vi "Write ImageDescription to tiff string.vi"(8 "error in":errorcluster, 10 "Tiff image (unsigned byte array)":u8[](array[numeric]), 11 "ImageDescription string\n(must be at least 5 char long)":string) -> (0 "error out":errorcluster, 2 "Tiff file out (unsigned byte array)":u8[](array[numeric]))   [LabVIEW 2015, in "Tiff reader.lvlib"]
doc: "This .vi adds metadata to the tiff file (represented as a string)."
uses:
  Tiff reader.lvlib
  FieldTypes.ctl
  IFD Entry.ctl
panel:
  out "Insert tag before inserting data?":bool
  out "Directories out 2":T1[](array[typedef])
  out "Byte stream offset\nwhere tag should have been":u32
  out "Directories in":T1[](array[typedef])
  out "Val/Offs":u32
  out "Time elapsed (ms)":u32
  out "Tag already exists?":bool
  out "Tag for metadata":T1
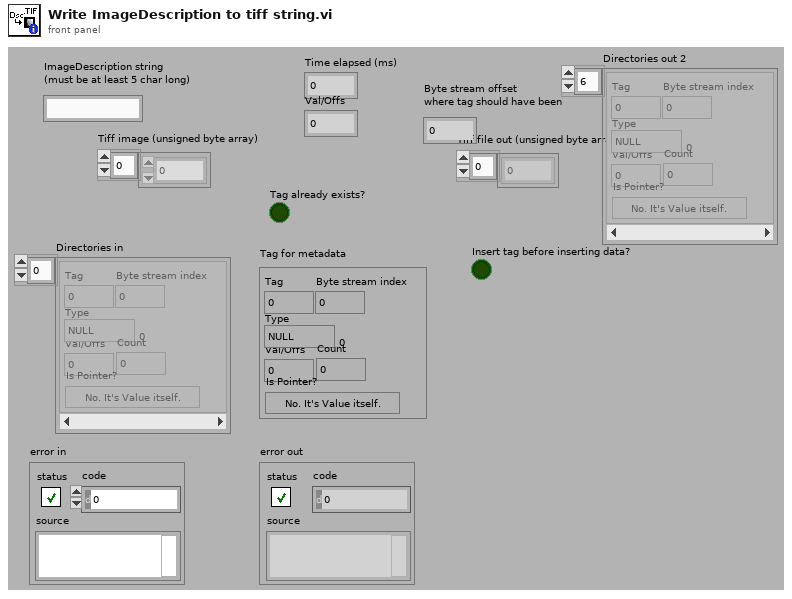
[diagram p1: front panel]
types:
  T1 = typedef "Tiff reader.lvlib/IFD Entry.ctl" = cluster{"Tag":u16, "Type":T2, "Count":u32, "Val/Offs":u32, "Is Pointer?":bool, "Byte stream index":i32}
  T2 = typedef "Tiff reader.lvlib/FieldTypes.ctl" = enum16{"NULL", "U8", "ASCII7", "U16", "U32", "RATIONAL", "SByte(I8)", "Undef(8Bit)", "I16", "I32", "SRat(4B:4B)", "SGL(4Byte)", "DBL(8Byte)"}
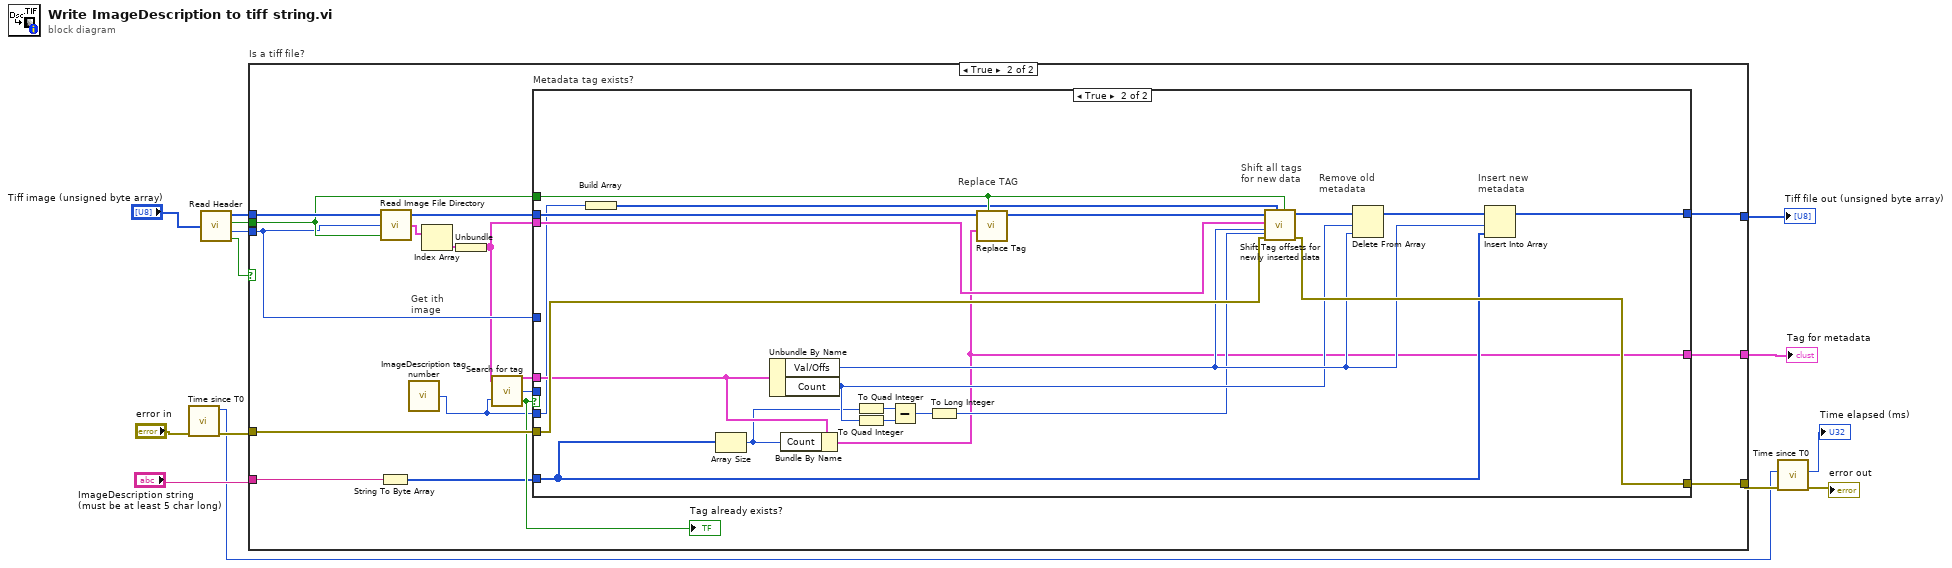
[diagram p0: block diagram]
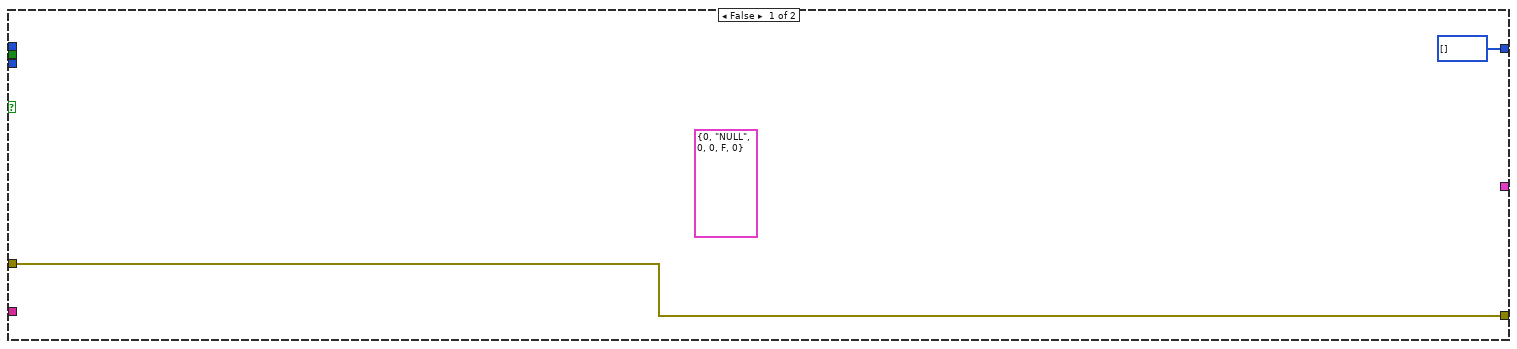
[diagram p2: hidden frame]
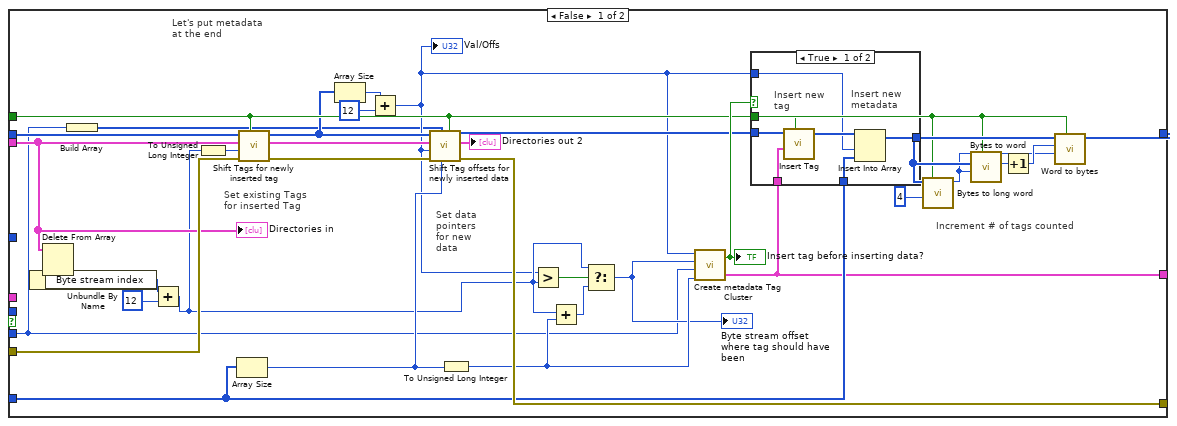
[diagram p3: hidden frame]
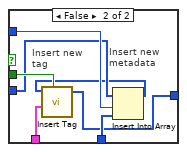
[diagram p4: hidden frame]
diagram:
  n1 = call "Time since T0.vi"("error in (no error)"="error in") -> ("error out"=w7:errorcluster, "current ms"=w3:u32)  [unwired: 2 in, 3 out]
  n2 = call "Read Header.vi"("TIFF Data in"="Tiff image (unsigned byte array)") -> ("TIFF Data out"=w13:u8[], "Litt/BigEnd"=w12:bool, "ImFileDirectOffs"=w14:u32, "IsTIFF?"=w11:bool)
  n3 = case "Is a tiff file?" shown="True" w11 {
    tunnel: w14 -> [_ w27]
    tunnel: w13 -> [_ w29]
    tunnel: [u8[] [] ("Image Data Out") w18] -> w9
    tunnel: w12 -> [_ w28]
    tunnel: "ImageDescription string\n(must be at least 5 char long)" -> [_ w33]
    tunnel: [_ w32] -> w2
    tunnel: w7 -> [w16 w31]
    tunnel: [w16 w30] -> w6
    frame False {
      (unwired) T1 {"Tag"=0, "Type"=enum."NULL", "Count"=0, "Val/Offs"=0, "Is Pointer?"=FALSE, "Byte stream index"=0} ("Tag found")
    }
    frame True {
      # "Get ith\nimage"
      n4 = String To Byte Array(string=w33) -> (unsigned byte array=w21:u8[])
      n5 = call "Read Image File Directory.vi"("Litt/BigEnd"=w28, "Im_File_Dir Offs"=w27, "Image Data in"=w29) -> ("Directories"=w26:cluster{"Tags":T1[]}[], "Image Data out"=w23:u8[])  [unwired: 1 out]
      n6 = call "ImageDescription tag number.vi"() -> ("ImageDescription"=w17:u16)
      n7 = Index Array(array=w26) -> (element=w20:cluster{"Tags":T1[]})  [unwired: 1 in]
      n8 = Unbundle(w20) -> ("Tags"=w19:T1[])
      n9 = call "Search for tag.vi"("Directory"=w19, "Tag"=w17) -> ("Tag found"=w25:T1, "Byte stream offset\nwhere tag should be"=w22:i32, "Tag exists?"=w24:bool)
      "Tag already exists?" <- w24
      n10 = case "Metadata tag exists?" shown="True" w24 {
        tunnel: w25 -> [_ w99]
        tunnel: w21 -> [w65 w98]
        tunnel: w23 -> [w64 w93]
        tunnel: w28 -> [w54 w84]
        tunnel: w19 -> [w45 w97]
        tunnel: w22 -> [_ _]
        tunnel: [w39 w85] -> w18
        tunnel: w17 -> [w35 w83]
        tunnel: [w62 w86] -> w32
        tunnel: w31 -> [w67 w102]
        tunnel: [w66 w101] -> w30
        tunnel: w27 -> [_ _]
        frame False {
          # "Increment # of tags counted"
          # "Set data \npointers\nfor new \ndata"
          # "Set existing Tags\nfor inserted Tag"
          # "Let's put metadata \nat the end"
          n11 = Delete From Array(array=w45) -> (deleted portion=w44:T1)  [unwired: 2 in, 1 out]
          n12 = Unbundle By Name(w44) -> ("Byte stream index"=w43:i32)
          n13 = Build Array(w35) -> (w34:u16[])
          n14 = Add(x=w43, y=12) -> (x+y=w41:i32)
          n15 = To Unsigned Long Integer(number=w41) -> (unsigned 32bit integer=w63:u32)
          n16 = Array Size(array=w65) -> (size(s)=w57:i32)
          n17 = call "Shift Tags for newly inserted tag.vi"("Litt/BigEnd"=w54, "error in"=w67, "Byte stream offset\nwhere new tag added"=w63, "Directories"=w45, "Image Data"=w64) -> ("error out"=w49:errorcluster, "Directories out"=w48:T1[], "Image Data Out"=w47:u8[])  [unwired: 1 in, 1 out]
          n18 = Array Size(array=w47) -> (size(s)=w37:i32)
          n19 = Add(x=w37, y=12) -> (x+y=w36:i32)
          "Val/Offs" <- w36
          n20 = call "Shift Tag offsets for newly inserted data.vi"("Litt/BigEnd"=w54, "Amount of data added\n(<0 means # of data bytesremoved)"=w57, "Ignore Tags"=w34, "error in"=w49, "Byte stream offset\nwhere new data added"=w36, "Directories"=w48, "Image Data"=w47) -> ("error out"=w66:errorcluster, "Directories out"=→"Directories out 2":T1[], "Image Data Out"=w55:u8[])  [unwired: 1 out]
          n21 = To Unsigned Long Integer(number=w57) -> (unsigned 32bit integer=w52:u32)
          n22 = Greater?(x=w36, y=w41) -> (0:w53:bool)
          n23 = Add(x=w41, y=w52) -> (x+y=w51:u32)
          n24 = Select(t=w41, s=w53, f=w51) -> (s? t:f=w50:u32)
          "Byte stream offset\nwhere tag should have been" <- w50
          n25 = call "Create metadata Tag Cluster.vi"("Count"=w52, "Tag to store\nmetadata in\n(ImageID tag)"=w35, "Byte stream offset\nwhere tag should have been"=w50, "Byte stream offset\nwhere data should be"=w36) -> ("Cluster"=w62:T1, "Insert tag before inserting data?"=w56:bool)
          "Insert tag before inserting data?" <- w56
          n26 = case shown="True" w56 {
            tunnel: w65 -> [w74 w81]
            tunnel: w55 -> [w73 w77]
            tunnel: w36 -> [w71 w80]
            tunnel: w62 -> [w70 w79]
            tunnel: [w69 w75] -> w58
            tunnel: w54 -> [w68 w78]
            frame True {
              # "Insert new \ntag"
              # "Insert new \nmetadata"
              n27 = call "Insert Tag.vi"("Image Data in"=w73, "Cluster"=w70, "Litt/BigEnd"=w68) -> ("Image Data Out"=w72:u8[])  [unwired: 4 out]
              n28 = Insert Into Array(array=w72, index=w71, new element=w74) -> (w69:u8[])
            }
            frame False {
              # "Insert new \ntag"
              # "Insert new \nmetadata"
              n29 = Insert Into Array(array=w77, index=w80, new element=w81) -> (w76:u8[])
              n30 = call "Insert Tag.vi"("Image Data in"=w76, "Cluster"=w79, "Litt/BigEnd"=w78) -> ("Image Data Out"=w75:u8[])  [unwired: 4 out]
            }
          }
          n31 = call "Bytes to long word.vi"("Litt/BigEnd"=w54, "Index"=4, "Image Data in"=w58) -> ("U32"=w40:u32)  [unwired: 6 out]
          n32 = call "Bytes to word.vi"("Litt/BigEnd"=w54, "Index"=w40, "Image Data in"=w58) -> ("Word"=w61:u16)  [unwired: 1 in, 5 out]
          n33 = Increment(x=w61) -> (x+1=w60:u16)
          n34 = call "Word to bytes.vi"("Litt/BigEnd"=w54, "Index"=w40, "Word"=w60, "Image Data in"=w58) -> ("Image Data out"=w39:u8[])  [unwired: 5 out]
          "Directories in" <- w45
        }
        frame True {
          # "Shift all tags\nfor new data"
          # "Replace TAG"
          # "Insert new \nmetadata"
          # "Remove old \nmetadata"
          n35 = Build Array(w83) -> (w82:u16[])
          n36 = Array Size(array=w98) -> (size(s)=w90:i32)
          n37 = Unbundle By Name(w99) -> ("Val/Offs"=w96:u32, "Count"=w91:u32)
          n38 = Bundle By Name(cluster=w99, "Count"=w90) -> (w86:T1)
          n39 = To Quad Integer(1:w90) -> (0:w89:i64)
          n40 = To Quad Integer(1:w91) -> (0:w92:i64)
          n41 = Subtract(x=w89, y=w92) -> (x-y=w88:i64)
          n42 = To Long Integer(number=w88) -> (32bit integer=w87:i32)
          n43 = call "Replace Tag.vi"("Litt/BigEnd"=w84, "Tag"=w86, "Image Data in"=w93) -> ("Image Data Out"=w94:u8[])  [unwired: 3 in, 2 out]
          n44 = call "Shift Tag offsets for newly inserted data.vi"("Litt/BigEnd"=w84, "Amount of data added\n(<0 means # of data bytesremoved)"=w87, "Ignore Tags"=w82, "error in"=w102, "Byte stream offset\nwhere new data added"=w96, "Directories"=w97, "Image Data"=w94) -> ("error out"=w101:errorcluster, "Image Data Out"=w95:u8[])  [unwired: 2 out]
          n45 = Delete From Array(array=w95, length=w91, index=w96) -> (array with subset deleted=w100:u8[])  [unwired: 1 out]
          n46 = Insert Into Array(array=w100, index=w96, new element=w98) -> (w85:u8[])
        }
      }
    }
  }
  "Tiff file out (unsigned byte array)" <- w9
  "Tag for metadata" <- w2
  n47 = call "Time since T0.vi"("error in (no error)"=w6, "T0 millisecond timer value"=w3) -> ("error out"=→"error out":errorcluster, "Time elapsed (ms)"=→"Time elapsed (ms)":u32)  [unwired: 1 in, 3 out]
